vi "Select Product.vi"(7 "Products in":T2, 8 "error in (no error)":errorcluster, 11 "Product_Data in":T1[](array[typedef])) -> (0 "error out":errorcluster, 1 "Product":T1, 2 "String":string, 3 "Product_Data out":T1[](array[typedef]))   [LabVIEW 2026]
uses:
  controls/Product.ctl
  controls/Products Enum.ctl
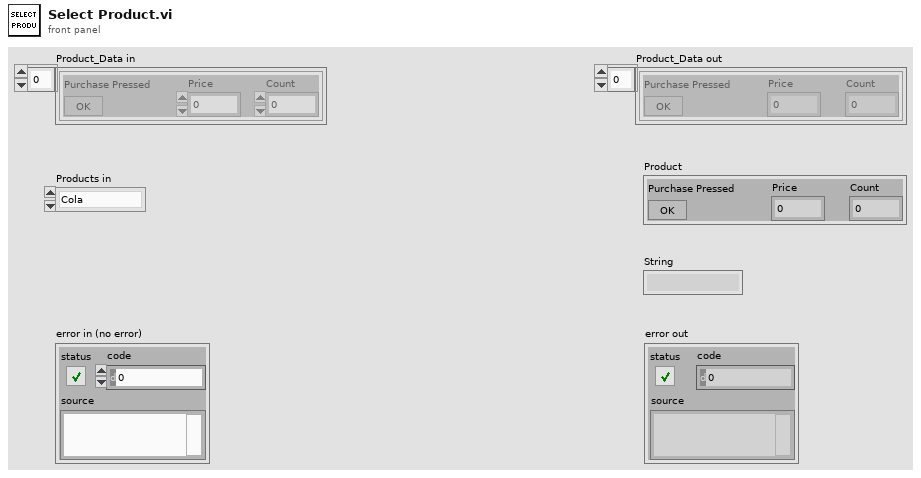
[diagram p1: front panel]
types:
  T1 = typedef "Product.ctl" = cluster{"Purchase Pressed":bool, "Price":dbl, "Count":i32}
  T2 = typedef "Products Enum.ctl" = enum16{"Cola", "Chips", "Candy"}
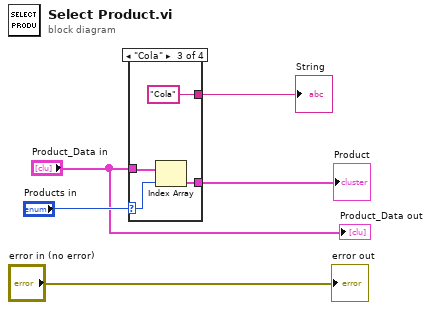
[diagram p0: block diagram]
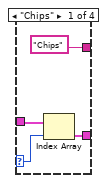
[diagram p2: hidden frame]
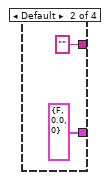
[diagram p3: hidden frame]
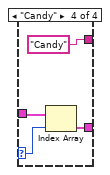
[diagram p4: hidden frame]
diagram:
  n1 = case shown="\"Cola\"" "Products in" {
    selector: "Products in" -> [w8 _ w14 w18]
    tunnel: [w7 T1 {"Purchase Pressed"=FALSE, "Price"=0.0, "Count"=0} ("Candy") w13 w17] -> w3
    tunnel: "Product_Data in" -> [w9 _ w15 w19]
    tunnel: ["Chips" "" "Cola" "Candy"] -> w5
    frame "Chips" {
      n2 = Index Array(array=w9, index=w8) -> (element=w7:T1)
    }
    frame Default {
    }
    frame "Cola" {
      n3 = Index Array(array=w15, index=w14) -> (element=w13:T1)
    }
    frame "Candy" {
      n4 = Index Array(array=w19, index=w18) -> (element=w17:T1)
    }
  }
  "String" <- w5
  "Product" <- w3
  "error out" <- "error in (no error)"
  "Product_Data out" <- "Product_Data in"
